vi "MouseDownEventHandler.vi"(4 "Mouse":T1, 5 "initialized MDF 2":T2[](array[typedef]) {"Latitude (waypoint)" format="%#_8g"; "Longitude  (waypoint)" format="%#_8g"}, 6 "Way Point Index":i32, 7 "MissionDefFile":picture, 8 "RobotSpeed_Leg":dbl, 9 "Behavior":T3(ring)) -> (0 "new picture":picture, 1 "initialized MDF":T2[](array[typedef]) {"Latitude (waypoint)" format="%#_8g"; "Longitude  (waypoint)" format="%#_8g"}, 2 "MDFile":T2 {"Latitude (waypoint)" format="%#_8g"; "Longitude  (waypoint)" format="%#_8g"}, 3 "Numeric":i32)   [LabVIEW 2010]
uses:
  6-OCU Neurons/MDF LatLong.ctl
  <vilib>/Utility/miscctls.llb/LVMouseTypeDef.ctl
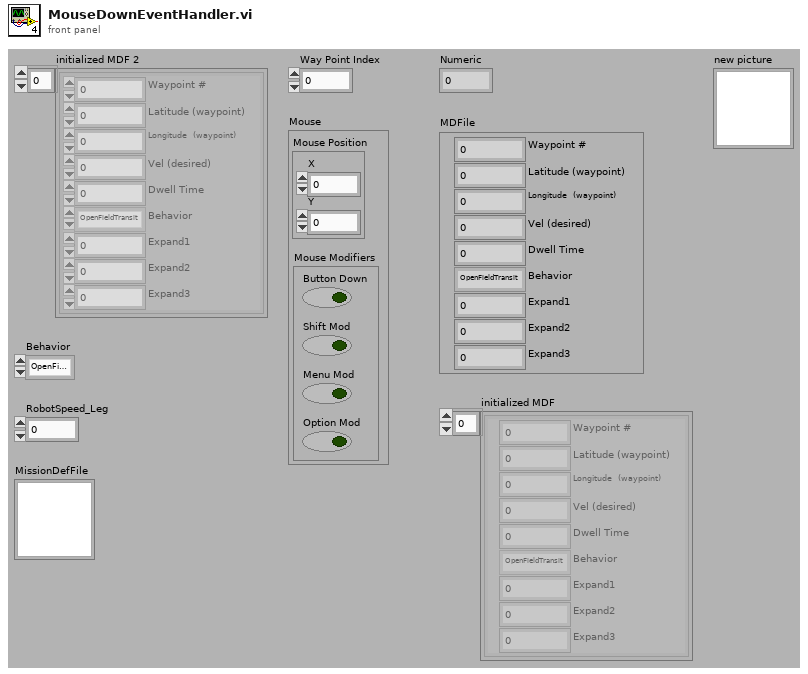
[diagram p1: front panel]
types:
  T1 = typedef "LVMouseTypeDef.ctl" = cluster{"Mouse Position":cluster{"X":i32, "Y":i32}, "Mouse Modifiers":cluster{"Button Down":bool, "Shift Mod":bool, "Menu Mod":bool, "Option Mod":bool}}
  T2 = typedef "MDF LatLong.ctl" = cluster{"Waypoint #":dbl, "Latitude (waypoint)":ext, "Longitude  (waypoint)":ext, "Vel (desired)":dbl, "Dwell Time":dbl, "Behavior":enum16{"OpenFieldTransit", "WallFollow", "LaneFollow", "ManualMode"}, "Expand1":dbl, "Expand2":dbl, "Expand3":dbl}
  T3 = enum16{"OpenFieldTransit", "WallFollow", "LaneFollow", "ManualMode"}
  T4 = cluster{"Width":u16, "Style":enum32{"Solid", "Dash", "Dot", "DashDot", "DashDotDot"}}
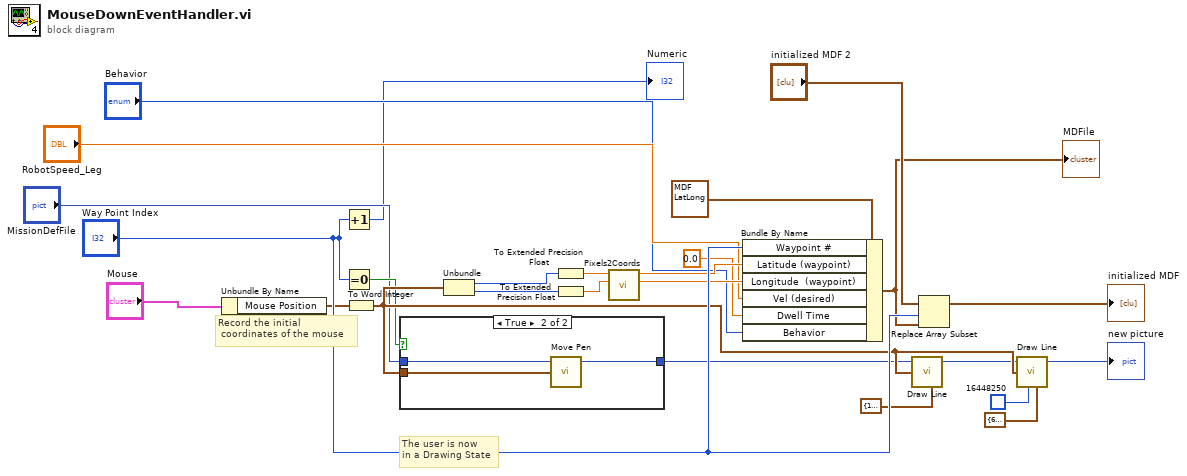
[diagram p0: block diagram]
diagram:
  # "Record the initial\n coordinates of the mouse"
  # "The user is now\nin a Drawing State"
  n1 = Unbundle By Name("Mouse") -> ("Mouse Position"=w3:cluster{"X":i32, "Y":i32})
  n2 = Increment(x="Way Point Index") -> (x+1=→"Numeric":i32)
  n3 = Equal To 0?(x="Way Point Index") -> (x = 0?=w20:bool)
  n4 = To Word Integer(number=w3) -> (16bit integer=w22:cluster{"X":i16, "Y":i16})
  n5 = case shown="True" w20 {
    tunnel: [w27 w30] -> w10
    tunnel: w22 -> [_ w29]
    tunnel: "MissionDefFile" -> [w27 w28]
    frame False {
    }
    frame True {
      n6 = call <vilib>:"Move Pen.vi"("new position"=w29, "picture"=w28) -> ("new picture"=w30:picture)  [unwired: 3 in]
    }
  }
  n7 = Unbundle(w22) -> ("X"=w6:i16, "Y"=w7:i16)
  n8 = To Extended Precision Float(1:w6) -> (0:w16:ext)
  n9 = To Extended Precision Float(1:w7) -> (0:w17:ext)
  n10 = call "Pixels2Coords.vi"("Y (pixels)"=w17, "X (pixels)"=w16) -> ("Latitude"=w19:ext, "Longtitude"=w18:ext)  [unwired: 8 in]
  n11 = Bundle By Name(cluster=T2 {"Waypoint #"=0.0, "Latitude (waypoint)"=0.0, "Longitude  (waypoint)"=0.0, "Vel (desired)"=0.0, "Dwell Time"=0.0, "Behavior"=enum."OpenFieldTransit", "Expand1"=0.0, "Expand2"=0.0, "Expand3"=0.0} ("MDFile"), "Waypoint #"="Way Point Index", "Latitude (waypoint)"=w18, "Longitude  (waypoint)"=w19, "Vel (desired)"="RobotSpeed_Leg", "Dwell Time"=0.0, "Behavior"="Behavior") -> (w5:T2)
  "MDFile" <- w5
  n12 = call <vilib>:"Draw Line.vi"("picture"=w10, "end point"=w22, "pen"=T4 {"Width"=1, "Style"=enum."Dot"}) -> ("new picture"=w21:picture)  [unwired: 6 in]
  n13 = Replace Array Subset(array="initialized MDF 2", new element=w5, index="Way Point Index") -> (→"initialized MDF":T2[])
  n14 = call <vilib>:"Draw Line.vi"("picture"=w21, "end point"=w22, "color(black)"=u32 16448250, "pen"=T4 {"Width"=6, "Style"=enum."Solid"}) -> ("new picture"=→"new picture":picture)  [unwired: 5 in]
